vi "test.Create.AddOrderLong.vi"(11 "AddOrderLong.Parameters":T1={"Time Offset"=447000, "Order Id"="ORID0001", "Quantity"=20000, "Symbol"="AAPL", "Side Indicator"="B", "Price"=0.905}) -> (3 "Passed":bool)   [LabVIEW 2022 SP3]
uses:
  AddOrder/AddOrderLong.Parameters.ctl
  AddOrder/AddOrderLong.lvclass
panel:
  out "x = y?":bool[](array[boolean])
  out "Python.Bytes.Out":u8[](array[numeric]) format="%.0x"
  out "LabVIEW.Bytes.Out":u8[](array[numeric]) format="%.0x"
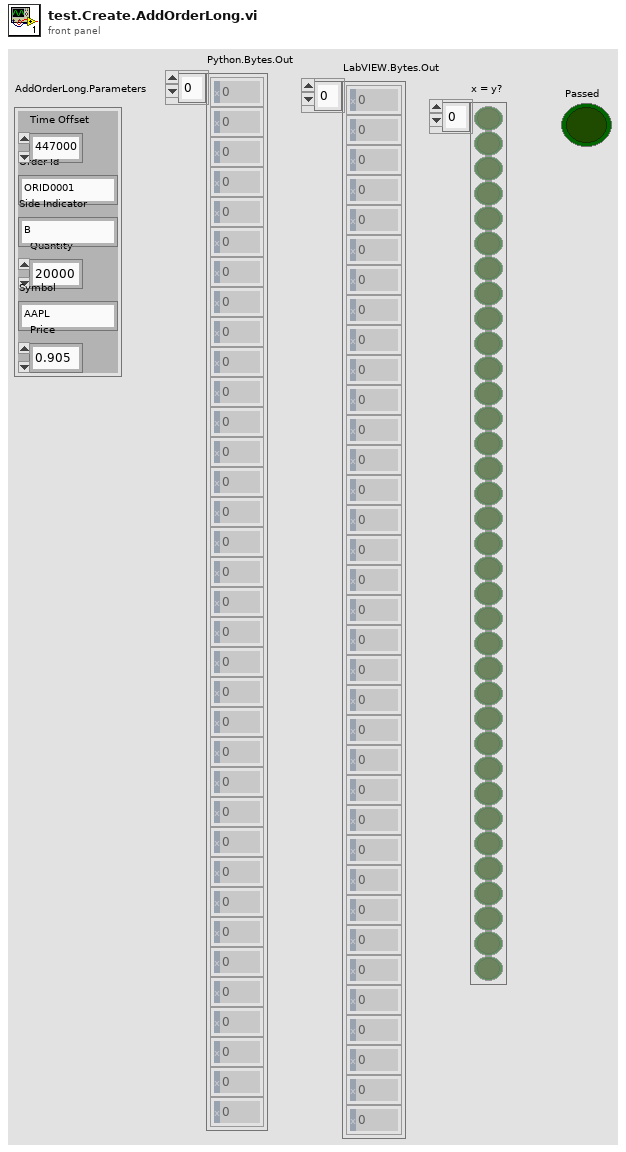
[diagram p1: front panel]
types:
  T1 = typedef "AddOrderLong.lvclass/AddOrderLong.Parameters.ctl" = cluster{"Time Offset":u32, "Order Id":string, "Quantity":u32, "Symbol":string, "Side Indicator":string, "Price":dbl}
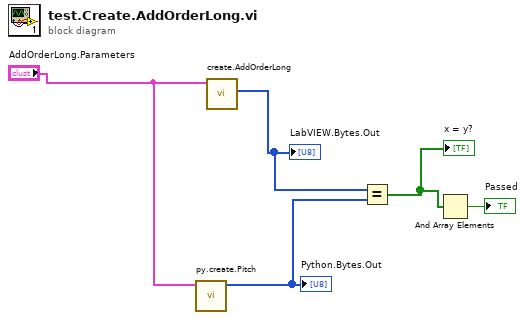
[diagram p0: block diagram]
diagram:
  n1 = call "py.create.Pitch.vi"("Parameters"="AddOrderLong.Parameters") -> ("bytes"=w5:u8[])  [unwired: 9 in, 1 out]
  "Python.Bytes.Out" <- w5
  n2 = call "create.AddOrderLong.vi"("AddOrderLong.Parameters"="AddOrderLong.Parameters") -> ("Bytes.Out"=w3:u8[])  [unwired: 9 in, 1 out]
  "LabVIEW.Bytes.Out" <- w3
  n3 = Equal?(x=w3, y=w5) -> (x = y?=w4:bool[])
  "x = y?" <- w4
  n4 = And Array Elements(Boolean array=w4) -> (logical AND=→"Passed":bool)
